vi "emi_Is FPGA.vi"(9 "error in (no error)":errorcluster) -> (8 "FPGA?":bool, 10 "error out":errorcluster)   [LabVIEW 2010]
doc: "Returns true if vi is running on an FPGA target.\n\nDoes not include error terminals to maximise performance.\n\nSubroutine"
panel:
  # "conditional disable klart raskes.\nFB er ikke langt etter"
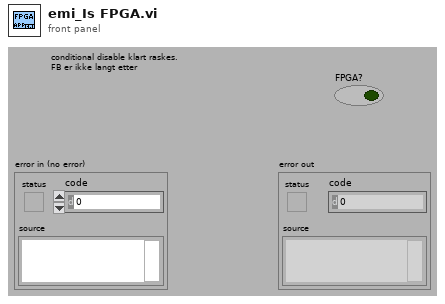
[diagram p1: front panel]
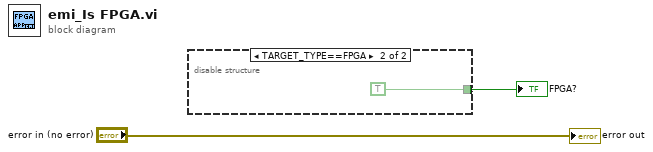
[diagram p0: block diagram]
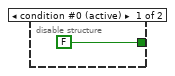
[diagram p2: hidden frame]
diagram:
  n1 = disable-structure shown="TARGET_TYPE==FPGA" {
    disable-tunnel: [FALSE TRUE ("Boolean")] -> w2
    frame condition #0 (active) {
    }
    frame condition #1 {
    }
  }
  "FPGA?" <- w2
  "error out" <- "error in (no error)"
